vi "Read Part ID.vi"(8 "error in (no error)":errorcluster, 11 "Thermistor in":refnum<class "Thermistor.lvclass">) -> (0 "error out":errorcluster, 2 "Part ID":string, 3 "Thermistor out":refnum<class "Thermistor.lvclass">)   [LabVIEW 2024, in "Thermistor.lvclass"]
uses:
  Thermistor.lvclass
  Thermistor.lvclass/Thermistor.ctl
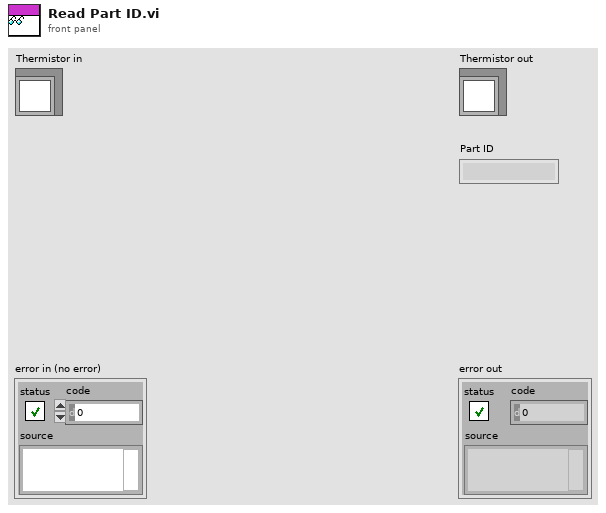
[diagram p1: front panel]
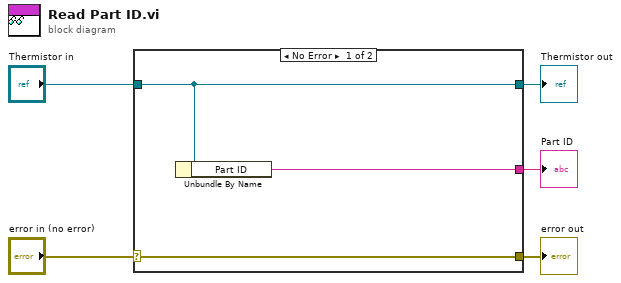
[diagram p0: block diagram]
diagram:
  n1 = case shown="No Error" "error in (no error)" {
    selector: "error in (no error)" -> [w8 w9]
    tunnel: [w8 w9] -> w4
    tunnel: [w7 w10] -> w2
    tunnel: "Thermistor in" -> [w7 w10]
    tunnel: [w6 _] -> w1
    frame No Error {
      n2 = Unbundle By Name(w7) -> ("Part ID"=w6:string)
    }
    frame Error {
    }
  }
  "error out" <- w4
  "Thermistor out" <- w2
  "Part ID" <- w1
